vi "Utility Read Modbus Address DataType.vi"(0 "VISA resource name":refnum<visa-resource-name>, 5 "Data Type":string[][](array[string]), 9 "Register Address (0)":dbl, 11 "error in (no error)":errorcluster) -> (4 "VISA resource name out":refnum<visa-resource-name>, 6 "Float32 (T)":bool, 10 "Index of Register Address":i32, 15 "error out":errorcluster)   [LabVIEW 2010, in "Eurotherm 32xx Series.lvlib"]
doc: "This VI reads the Data type of a Register Address (also known as Parameter Modbus Address)."
uses:
  <instrlib>/Eurotherm 32xx Series/Eurotherm 32xx Series.lvlib
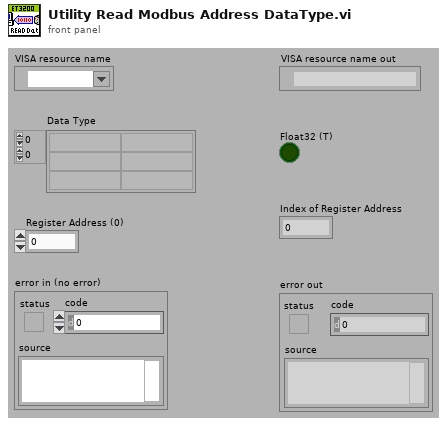
[diagram p1: front panel]
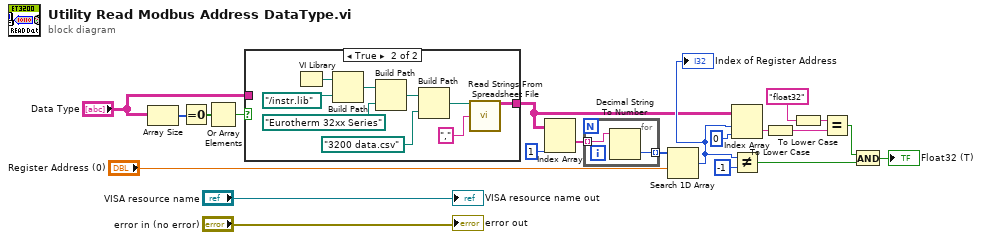
[diagram p0: block diagram]
diagram:
  n1 = Array Size(array="Data Type") -> (size(s)=w8:i32[])
  n2 = Equal To 0?(x=w8) -> (x = 0?=w7:bool[])
  n3 = Or Array Elements(Boolean array=w7) -> (logical OR=w6:bool)
  n4 = case shown="True" w6 {
    tunnel: [w22 w31] -> w3
    tunnel: "Data Type" -> [w22 _]
    frame False {
    }
    frame True {
      n5 = VI Library() -> (path=w28:path)
      n6 = Build Path(base path=w28, name or relative path=path "../instr.lib" ("Relative path (.)")) -> (appended path=w26:path)
      n7 = Build Path(base path=w26, name or relative path=path "Eurotherm 32xx Series") -> (appended path=w23:path)
      n8 = Build Path(base path=w23, name or relative path=path "3200 data.csv") -> (appended path=w24:path)
      n9 = call <instrlib>:"Read Strings From Spreadsheet File.vi"("file path (dialog if empty)"=w24, "Delimiter (Tab)"="," ("delimiter (Tab)")) -> ("All Rows"=w31:string[][])  [unwired: 9 in, 4 out]
    }
  }
  n10 = Index Array(array=w3, index (col)=1 ("disabled index (col)")) -> (element=w21:string[])  [unwired: 1 in]
  n11 = for {
    tunnel: w21 -> [w32] mode=indexing
    tunnel: [w33] -> w4 mode=indexing
    n12 = Decimal String To Number(string=w32) -> (number=w33:i32)  [unwired: 2 in, 1 out]
  }
  n13 = Search 1D Array(1D array=w4, element="Register Address (0)") -> (index of element=w17:i32)  [unwired: 1 in]
  "Index of Register Address" <- w17
  n14 = Index Array(array=w3, index (row)=w17, index (col)=0 ("disabled index (col)")) -> (element=w16:string)
  n15 = Not Equal?(x=w17, y=-1) -> (x != y?=w11:bool)
  n16 = To Lower Case(string=w16) -> (all lower case string=w15:string)
  n17 = To Lower Case(string="float32") -> (all lower case string=w13:string)
  n18 = Equal?(x=w13, y=w15) -> (x = y?=w12:bool)
  n19 = And(x=w12, y=w11) -> (x .and. y?=→"Float32 (T)":bool)
  "error out" <- "error in (no error)"
  "VISA resource name out" <- "VISA resource name"
